vi "Copy_SourceItem.vi"(7 "referencedNonLVTypeMembers in":T1[](array[typedef]), 8 "error in (no error)":errorcluster, 10 "AB_Build.lvclass":refnum<class "AB_Build.lvclass">, 11 "AB_Source_Exported_Assembly_VI in":refnum<class "AB_Source_Exported_Assembly_VI.lvclass">) -> (0 "error out":errorcluster, 1 "newFileFlags":T2, 2 "newFileInfo":T3, 3 "AB_Source_Exported_Assembly_VI out":refnum<class "AB_Source_Exported_Assembly_VI.lvclass">, 5 "referencedNonLVTypeMembers out":T1[](array[typedef]))   [LabVIEW 2020, in "AB_Source_Exported_Assembly_VI.lvclass"]
uses:
  <vilib>/AppBuilder/AB_Classes/Source/ExportedAssemblyVI/AB_Source_Exported_Assembly_VI.lvclass
  <vilib>/AppBuilder/AB_Classes/Build/AB_Build.lvclass
  <vilib>/AppBuilder/Engine/AB_Engine_New_File_Info.ctl
  <vilib>/AppBuilder/Engine/AB_Engine_New_File_Flags.ctl
  <vilib>/AppBuilder/AB_Source_Referenced_Libray_Files.ctl
  <vilib>/AppBuilder/AB_Classes/Source/VI/AB_Source_VI.lvclass
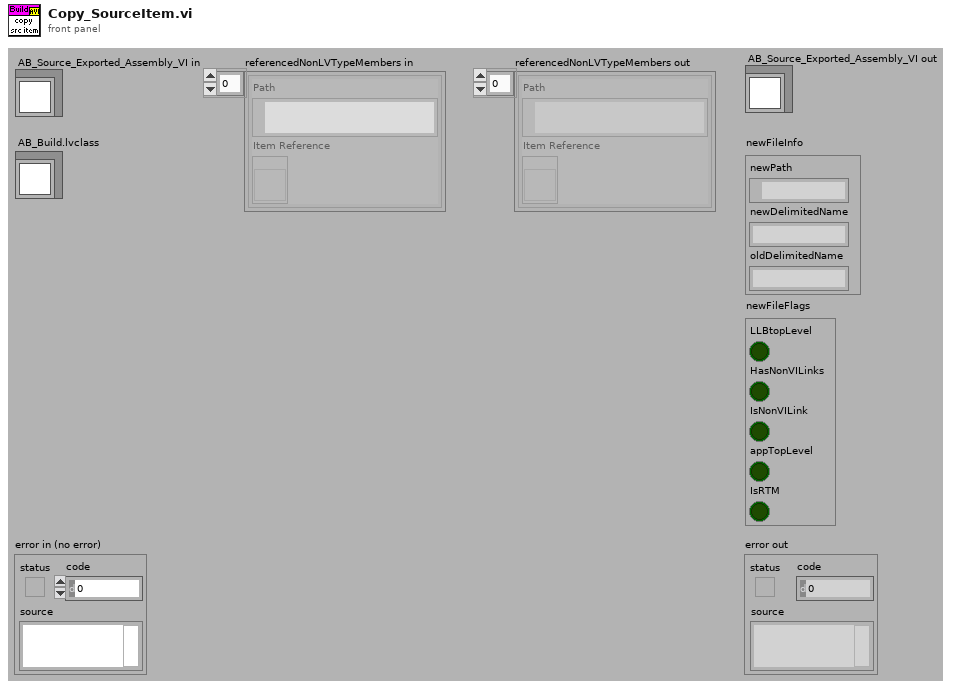
[diagram p1: front panel]
types:
  T1 = typedef "AB_Source_Referenced_Libray_Files.ctl" = cluster{"Path":path, "Item Reference":refnum<vi>}
  T2 = typedef "AB_Engine_New_File_Flags.ctl" = cluster{"LLBtopLevel":bool, "HasNonVILinks":bool, "IsNonVILink":bool, "appTopLevel":bool, "IsRTM":bool}
  T3 = typedef "AB_Engine_New_File_Info.ctl" = cluster{"newPath":path, "newDelimitedName":string, "oldDelimitedName":string}
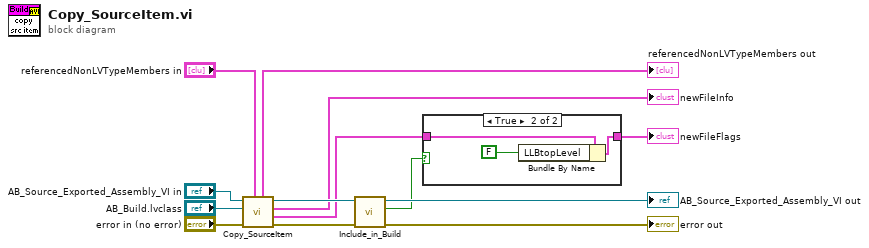
[diagram p0: block diagram]
diagram:
  n1 = call-parent "Copy_SourceItem.vi"("referencedNonLVTypeMembers in"="referencedNonLVTypeMembers in", "error in (no error)"="error in (no error)", "AB_Build.lvclass"="AB_Build.lvclass", "AB_Source_VI in"="AB_Source_Exported_Assembly_VI in") -> ("error out"=w6:errorcluster, "newFileFlags"=w2:T2, "newFileInfo"=→"newFileInfo":T3, "AB_Source_VI out"=w8:refnum<class "AB_Source_Exported_Assembly_VI.lvclass">, "referencedNonLVTypeMembers out"=→"referencedNonLVTypeMembers out":T1[])  [unwired: 3 out]
  n2 = call-dynamic "Include_in_Build.vi"("error in (no error)"=w6, "AB_Source in"=w8) -> ("error out"=→"error out":errorcluster, "includeInBuild"=w4:bool, "AB_Source out"=→"AB_Source_Exported_Assembly_VI out":refnum<class "AB_Source_Exported_Assembly_VI.lvclass">)  [unwired: 7 out]
  n3 = case shown="True" w4 {
    tunnel: w2 -> [w14 w17]
    tunnel: [w14 w16] -> w1
    frame False {
    }
    frame True {
      n4 = Bundle By Name(cluster=w17, "LLBtopLevel"=FALSE) -> (w16:T2)
    }
  }
  "newFileFlags" <- w1
